vi "7-3.vi"() -> ()   [LabVIEW 2017]
panel:
  in  "stop":bool
  in  "Tab Control":enum32{"Page 1", "Page 2", "Page 3", "Page 4"}(tab)
  out "sawtooth":dynamicdata(graph)
  out "square":dynamicdata(graph)
  out "triangle":dynamicdata(graph)
  out "sine":dynamicdata(graph)
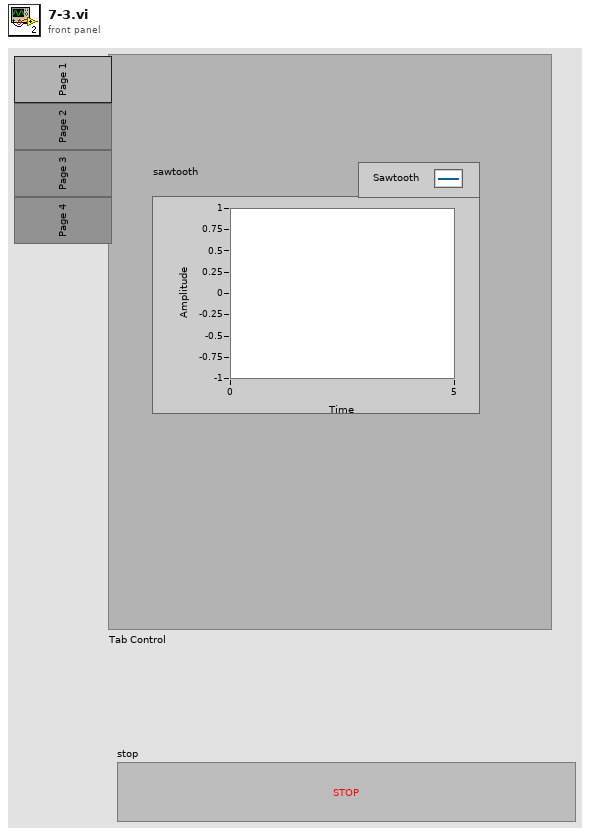
[diagram p1: front panel]
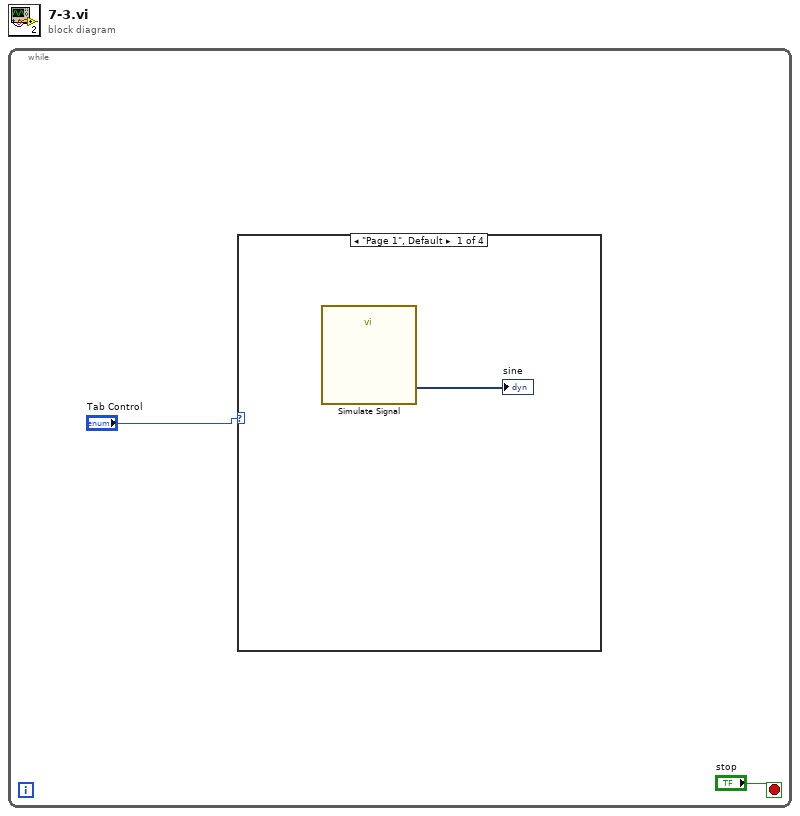
[diagram p0: block diagram]
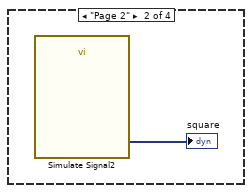
[diagram p2: hidden frame]
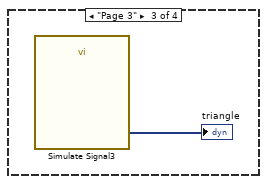
[diagram p3: hidden frame]
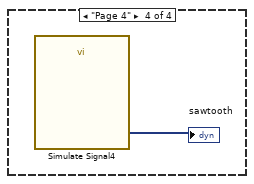
[diagram p4: hidden frame]
diagram:
  n1 = while {
    stop <- "stop" stop-if-true
    n2 = case shown="\"Page 1\", Default" "Tab Control" {
      frame "Page 1", Default {
        n3 = call "Simulate Signal"() -> ("Sawtooth"=→"sine":dynamicdata)  [unwired: 14 in, 1 out]
      }
      frame "Page 2" {
        n4 = call "Simulate Signal2"() -> ("Square"=→"square":dynamicdata)  [unwired: 14 in, 1 out]
      }
      frame "Page 3" {
        n5 = call "Simulate Signal3"() -> ("Triangle"=→"triangle":dynamicdata)  [unwired: 14 in, 1 out]
      }
      frame "Page 4" {
        n6 = call "Simulate Signal4"() -> ("Sine"=→"sawtooth":dynamicdata)  [unwired: 14 in, 1 out]
      }
    }
  }
